vi "FujiDelta Test.vi"() -> ()   [LabVIEW 2014]
uses:
  ALPHA5 RS485/typedefs/Port Selection Info.ctl
  GitHub/MyCode/Common/Delta Robot Kinematics/Delta Robot Param.ctl
  Delta Robot/Fuji Delta Robot.lvclass/Fuji Delta Robot.ctl
  ALPHA5 RS485/Classes/FujiMotor/FujiMotor.lvclass
  GitHub/MyCode/Common/Delta Robot Kinematics/Delta Robot Kinematics.lvclass
  Delta Robot/Fuji Delta Robot.lvclass
  ALPHA5 RS485/ALPHA5 RS485.lvlib
panel:
  out "end":bool
  in  "index":i32(ring) items=["X", "Y", "Z"]
  out "Waveform Chart 4":cluster{"Numeric":dbl, "X":dbl, "Numeric":dbl}(graph)
  out "sensed joints":dbl[](array[numeric])
  in  "Set Pos":bool
  in  "Position Cmd":cluster{"X":dbl, "Y":dbl, "Z":dbl} {"Z" scale=-0.8..-0.5; "Y" scale=-0.2..0.2; "X" scale=-0.2..0.2}
  out "Waveform Chart 3":cluster{"Slide":dbl, "ENC Pos":i32}(graph)
  out "Waveform Chart 2":cluster{"Slide":dbl, "ENC Pos":i32}(graph)
  in  "ON/OFF":bool[](array[boolean])=[FALSE, FALSE, FALSE]
  in  "Joints":dbl[](array[slide])=[0.0, 0.0, 0.0]
  in  "stop":bool
  in  "Inst Vel":i32=20000
  out "Waveform Chart":cluster{"Slide":dbl, "ENC Pos":i32}(graph)
  in  "Port Selection Info In":T1={"Port Name"="COM5", "Amplifier Num"=1, "Baud Rate"=38400, "Char Formation"=enum."0"} {"Baud Rate" items=["38400"=38400, "19200"=19200, "9600"=9600, "115200"=0]; "Amplifier Num" max=31}
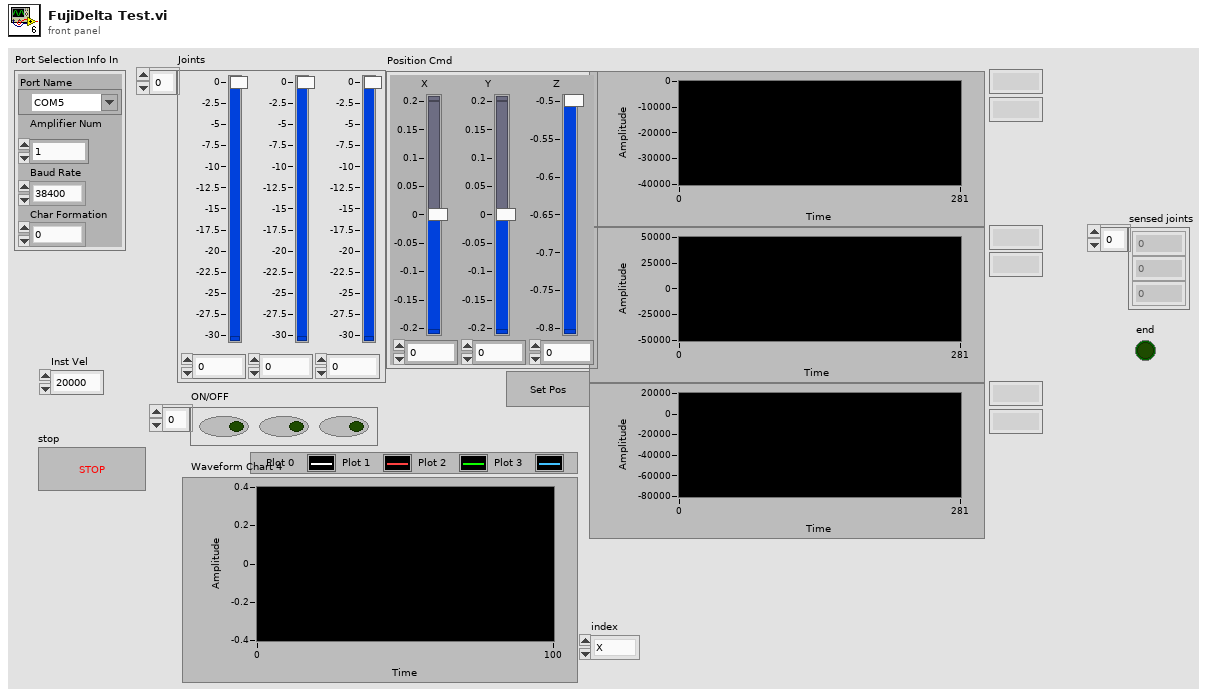
[diagram p1: front panel]
types:
  T1 = typedef "ALPHA5 RS485.lvlib/Port Selection Info.ctl" = cluster{"Port Name":refnum<visa-resource-name>, "Amplifier Num":u8, "Baud Rate":u32, "Char Formation":enum16{"0", "1", "2", "3", "4", "5"}}
  T2 = typedef "Delta Robot Kinematics.lvclass/Delta Robot Param.ctl" = cluster{"f":dbl, "e":dbl, "rf":dbl, "re":dbl}
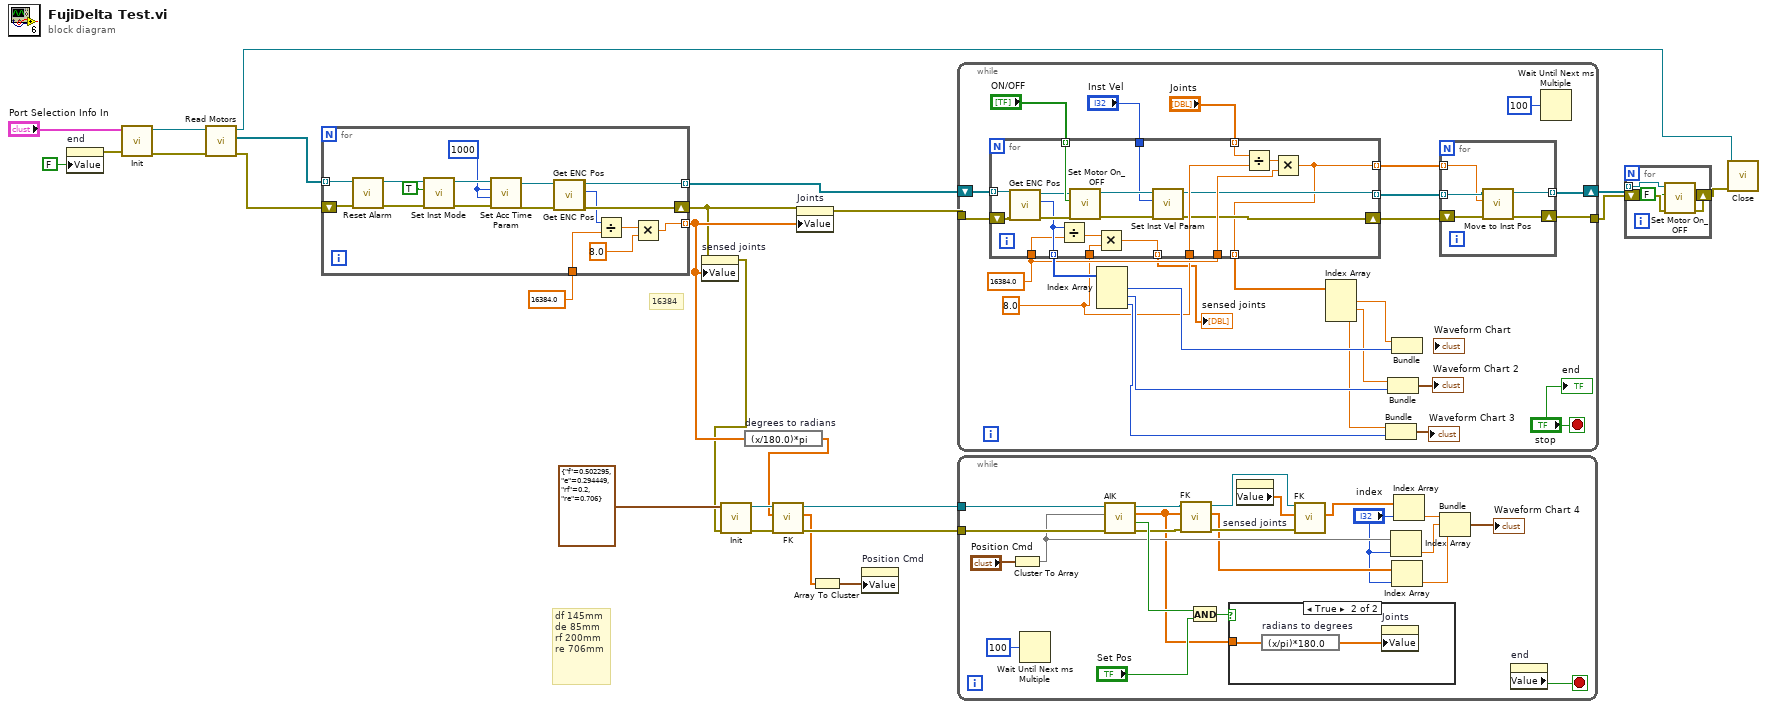
[diagram p0: block diagram]
diagram:
  # "df 145mm\nde 85mm\nrf 200mm \nre 706mm"
  # "16384"
  n1 = property on="end" class="Bool (strict)"("Value"=FALSE ("end")) -> (error out=w2:errorcluster)  [unwired: 2 in, 1 out]
  n2 = call "Init.vi"("error in (no error)"=w2, "Port Selection Info In"="Port Selection Info In") -> ("error out"=w23:errorcluster, "Fuji Delta out"=w24:refnum<class "Fuji Delta Robot.lvclass">)  [unwired: 8 in]
  n3 = call "Read Motors.vi"("error in (no error)"=w23, "Fuji Delta Robot in"=w24) -> ("error out"=w17:errorcluster, "Motors"=w16:refnum<class "FujiMotor.lvclass">[], "Fuji Delta Robot out"=w22:refnum<class "Fuji Delta Robot.lvclass">)  [unwired: 7 in]
  n4 = for {
    tunnel: [w37] -> w18 mode=indexing
    shift-right: [w35] -> w4
    shift-left: w17 -> [w32]
    tunnel: w16 -> [w31] mode=indexing
    tunnel: [w26] -> w5 mode=indexing
    tunnel: 16384.0 ("y") -> [w29]
    w39 = 1000 ("ACC Time")
    n5 = call "Reset Alarm.vi"("error in (no error)"=w32, "FujiMotor in"=w31) -> ("error out"=w33:errorcluster, "FujiMotor out"=w34:refnum<class "FujiMotor.lvclass">)  [unwired: 8 in]
    n6 = call "Set Inst Mode.vi"("error in (no error)"=w33, "ABS/INC"=TRUE, "FujiMotor in"=w34) -> ("error out"=w40:errorcluster, "FujiMotor out"=w41:refnum<class "FujiMotor.lvclass">)  [unwired: 7 in]
    n7 = call "Set Acc Time Param.vi"("error in (no error)"=w40, "DEC Time"=w39, "ACC Time"=w39, "FujiMotor in"=w41) -> ("error out"=w36:errorcluster, "FujiMotor out"=w38:refnum<class "FujiMotor.lvclass">)  [unwired: 6 in]
    n8 = call "Get ENC Pos.vi"("FujiMotor in"=w38) -> ()  [unwired: 8 in, 3 out]
    n9 = call "Get ENC Pos.vi"("error in (no error)"=w36, "FujiMotor in"=w38) -> ("error out"=w35:errorcluster, "ENC Pos"=w30:i32, "FujiMotor out"=w37:refnum<class "FujiMotor.lvclass">)  [unwired: 7 in]
    n10 = Divide(x=w30, y=w29) -> (x/y=w28:dbl)
    n11 = Multiply(x=w28, y=8.0) -> (x*y=w26:dbl)
  }
  n12 = property on="sensed joints" class="Arr (strict)"(error in=w4, "Value"=w5) -> (error out=w3:errorcluster)  [unwired: 1 in, 1 out]
  n13 = call "Init.vi"("error in (no error)"=w3, "Delta Param"=T2 {"f"=0.502295, "e"=0.294449, "rf"=0.2, "re"=0.706}) -> ("error out"=w12:errorcluster, "Delta Robot Kin"=w11:refnum<class "Delta Robot Kinematics.lvclass">)  [unwired: 8 in]
  n14 = expression code="(x/180.0)*pi" "degrees to radians"(w5) -> (w8:dbl[])
  n15 = call-dynamic "FK.vi"("error in (no error)"=w12, "joints"=w8, "Delta Robot Kinematics in"=w11) -> ("error out"=w9:errorcluster, "p"=w7:dbl[], "Delta Robot Kinematics out"=w10:refnum<class "Delta Robot Kinematics.lvclass">)  [unwired: 5 in, 1 out]
  n16 = property on="Joints" class="Arr (strict)"(error in=w4, "Value"=w5) -> (error out=w15:errorcluster)  [unwired: 1 in, 1 out]
  n17 = Array To Cluster(array=w7) -> (cluster=w6:cluster{"p[0]":dbl, "p[1]":dbl, "p[2]":dbl})
  n18 = property on="Position Cmd" class="Clust (strict)"("Value"=w6) -> ()  [unwired: 2 in, 2 out]
  n19 = while {
    tunnel: w15 -> [w65]
    tunnel: [w44] -> w20
    shift-right: [w46] -> w21
    shift-left: w18 -> [w66]
    stop <- "stop" stop-if-true
    w50 = 8.0 ("y")
    w51 = 16384.0 ("y")
    n20 = for {
      tunnel: "ON/OFF" -> [w92] mode=indexing
      tunnel: "Inst Vel" -> [w89]
      tunnel: [w75] -> w47 mode=indexing
      tunnel: w66 -> [w88] mode=indexing
      tunnel: [w73] -> w60 mode=indexing
      tunnel: [w82] -> w61 mode=indexing
      shift-right: [w74] -> w45
      shift-left: w65 -> [w87]
      tunnel: "Joints" -> [w84] mode=indexing
      tunnel: w51 -> [w81]
      tunnel: w51 -> [w80]
      tunnel: w50 -> [w78]
      tunnel: w50 -> [w77]
      tunnel: [w76] -> w49 mode=indexing
      tunnel: [w73] -> w43 mode=indexing
      n21 = call "Get ENC Pos.vi"("error in (no error)"=w87, "FujiMotor in"=w88) -> ("error out"=w86:errorcluster, "ENC Pos"=w82:i32, "FujiMotor out"=w85:refnum<class "FujiMotor.lvclass">)  [unwired: 7 in]
      n22 = Divide(x=w82, y=w81) -> (x/y=w79:dbl)
      n23 = call "Set Motor On_OFF.vi"("error in (no error)"=w86, "ON/OFF"=w92, "FujiMotor in"=w85) -> ("error out"=w91:errorcluster, "FujiMotor out"=w90:refnum<class "FujiMotor.lvclass">)  [unwired: 7 in]
      n24 = Multiply(x=w79, y=w78) -> (x*y=w76:dbl)
      n25 = call "Set Inst Vel Param.vi"("error in (no error)"=w91, "Inst Vel"=w89, "FujiMotor in"=w90) -> ("error out"=w74:errorcluster, "FujiMotor out"=w75:refnum<class "FujiMotor.lvclass">)  [unwired: 7 in]
      n26 = Divide(x=w84, y=w77) -> (x/y=w83:dbl)
      n27 = Multiply(x=w83, y=w80) -> (x*y=w73:dbl)
    }
    "sensed joints" <- w49
    n28 = Index Array(array=w61) -> (element #1=w58:i32, element #2=w56:i32, element #3=w54:i32)  [unwired: 3 in]
    n29 = Index Array(array=w60) -> (element #1=w59:dbl, element #2=w57:dbl, element #3=w55:dbl)  [unwired: 3 in]
    n30 = Bundle(w55, "ENC Pos"=w54) -> (→"Waveform Chart 3":cluster{dbl, "ENC Pos":i32})  [unwired: 1 in]
    n31 = Bundle(w57, "ENC Pos"=w56) -> (→"Waveform Chart 2":cluster{dbl, "ENC Pos":i32})  [unwired: 1 in]
    n32 = Bundle(w59, "ENC Pos"=w58) -> ()  [unwired: 1 in, 1 out]
    n33 = for {
      tunnel: w47 -> [w72] mode=indexing
      tunnel: [w71] -> w46 mode=indexing
      shift-right: [w69] -> w44
      shift-left: w45 -> [w70]
      tunnel: w43 -> [w68] mode=indexing
      n34 = call "Move to Inst Pos.vi"("error in (no error)"=w70, "Inst Pos"=w68, "FujiMotor in"=w72) -> ("error out"=w69:errorcluster, "FujiMotor out"=w71:refnum<class "FujiMotor.lvclass">)  [unwired: 7 in]
    }
    n35 = Wait Until Next ms Multiple(millisecond multiple=u32 100) -> ()  [unwired: 1 out]
    "end" <- "stop"
  }
  n36 = while {
    tunnel: w10 -> [w114]
    tunnel: w9 -> [w113]
    stop <- w94 stop-if-true
    n37 = Cluster To Array(cluster="Position Cmd") -> (array=w103:dbl[])
    n38 = Wait Until Next ms Multiple(millisecond multiple=u32 100) -> ()  [unwired: 1 out]
    n39 = call-dynamic "AIK.vi"("error in (no error)"=w113, "p"=w103, "Delta Robot Kinematics in"=w114) -> ("error out"=w106:errorcluster, "exist"=w109:bool, "joints"=w95:dbl[], "Delta Robot Kinematics out"=w107:refnum<class "Delta Robot Kinematics.lvclass">)  [unwired: 5 in]
    n40 = call-dynamic "FK.vi"("error in (no error)"=w106, "joints"=w95, "Delta Robot Kinematics in"=w107) -> ("error out"=w105:errorcluster, "p"=w102:dbl[], "Delta Robot Kinematics out"=w104:refnum<class "Delta Robot Kinematics.lvclass">)  [unwired: 5 in, 1 out]
    n41 = And(x=w109, y="Set Pos") -> (x .and. y?=w110:bool)
    n42 = case shown="True" w110 {
      tunnel: w95 -> [_ w116]
      frame False {
      }
      frame True {
        n43 = expression code="(x/pi)*180.0" "radians to degrees"(w116) -> (w115:dbl[])
        n44 = property on="Joints" class="Arr (strict)"("Value"=w115) -> ()  [unwired: 2 in, 2 out]
      }
    }
    n45 = property on="sensed joints" class="Arr (strict)"() -> ("Value"=w111:dbl[])  [unwired: 2 in, 2 out]
    n46 = call-dynamic "FK.vi"("error in (no error)"=w105, "joints"=w111, "Delta Robot Kinematics in"=w104) -> ("p"=w101:dbl[])  [unwired: 5 in, 3 out]
    n47 = Index Array(array=w103, index="index") -> (element=w98:dbl)
    n48 = Index Array(array=w102, index="index") -> (element=w97:dbl)
    n49 = Index Array(array=w101, index="index") -> (element=w99:dbl)
    n50 = Bundle("Numeric"=w99, "X"=w98, "Numeric"=w97) -> (→"Waveform Chart 4":cluster{"Numeric":dbl, "X":dbl, "Numeric":dbl})  [unwired: 1 in]
    n51 = property on="end" class="Bool (strict)"() -> ("Value"=w94:bool)  [unwired: 2 in, 2 out]
  }
  n52 = for {
    tunnel: w21 -> [w120] mode=indexing
    shift-right: [w118] -> w19
    shift-left: w20 -> [w119]
    n53 = call "Set Motor On_OFF.vi"("error in (no error)"=w119, "ON/OFF"=FALSE, "FujiMotor in"=w120) -> ("error out"=w118:errorcluster)  [unwired: 7 in, 1 out]
  }
  n54 = call "Close.vi"("error in (no error)"=w19, "Fuji Delta in"=w22) -> ()  [unwired: 9 in, 1 out]
